vi "AddFailure.vi"(7 "Time":dbl, 8 "error in (no error)":errorcluster, 9 "Failure":errorcluster, 10 "Test":refnum<class "Test.lvclass">, 11 "TestListener in":refnum<class "TestListener.lvclass">) -> (0 "error out":errorcluster, 3 "TestListener out":refnum<class "TestListener.lvclass">)   [LabVIEW 2019, in "TestListener.lvclass"]
doc: "A failure occurred."
uses:
  TestListener.lvclass
  Test/Test.lvclass
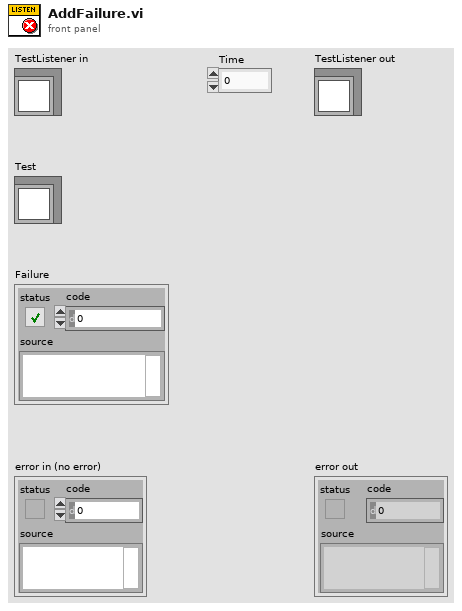
[diagram p1: front panel]
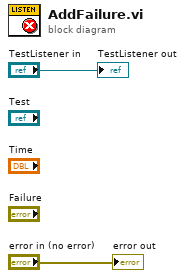
[diagram p0: block diagram]
diagram:
  "error out" <- "error in (no error)"
  "TestListener out" <- "TestListener in"
